vi "Revision Query.vi"(8 "error in (no error)":errorcluster, 11 "VISA resource name":refnum<visa-resource-name>) -> (0 "error out":errorcluster, 1 "Instrument Firmware Revision":string, 2 "Instrument Driver Revision":string, 3 "VISA resource name out":refnum<visa-resource-name>)   [LabVIEW 2025]
doc: "Queries the current instrument firmware revision and instrument driver revision.\n\nRefer to the Readme file for detailed driver information including modification history."
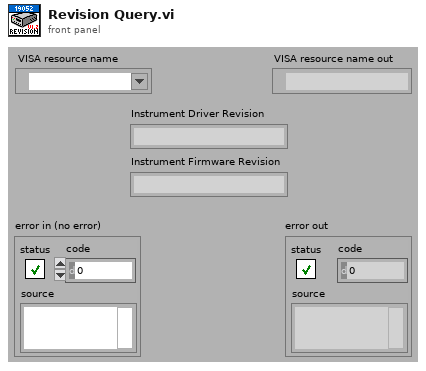
[diagram p1: front panel]
types:
  T1 = enum32{"invalid app kind", "Development System", "Run Time System", "Student Edition", "Embedded LabVIEW", "Evaluation", "Custom"}
  T2 = cluster{"Major":u16, "Minor":u16, "Fix":u16, "Build":u16}
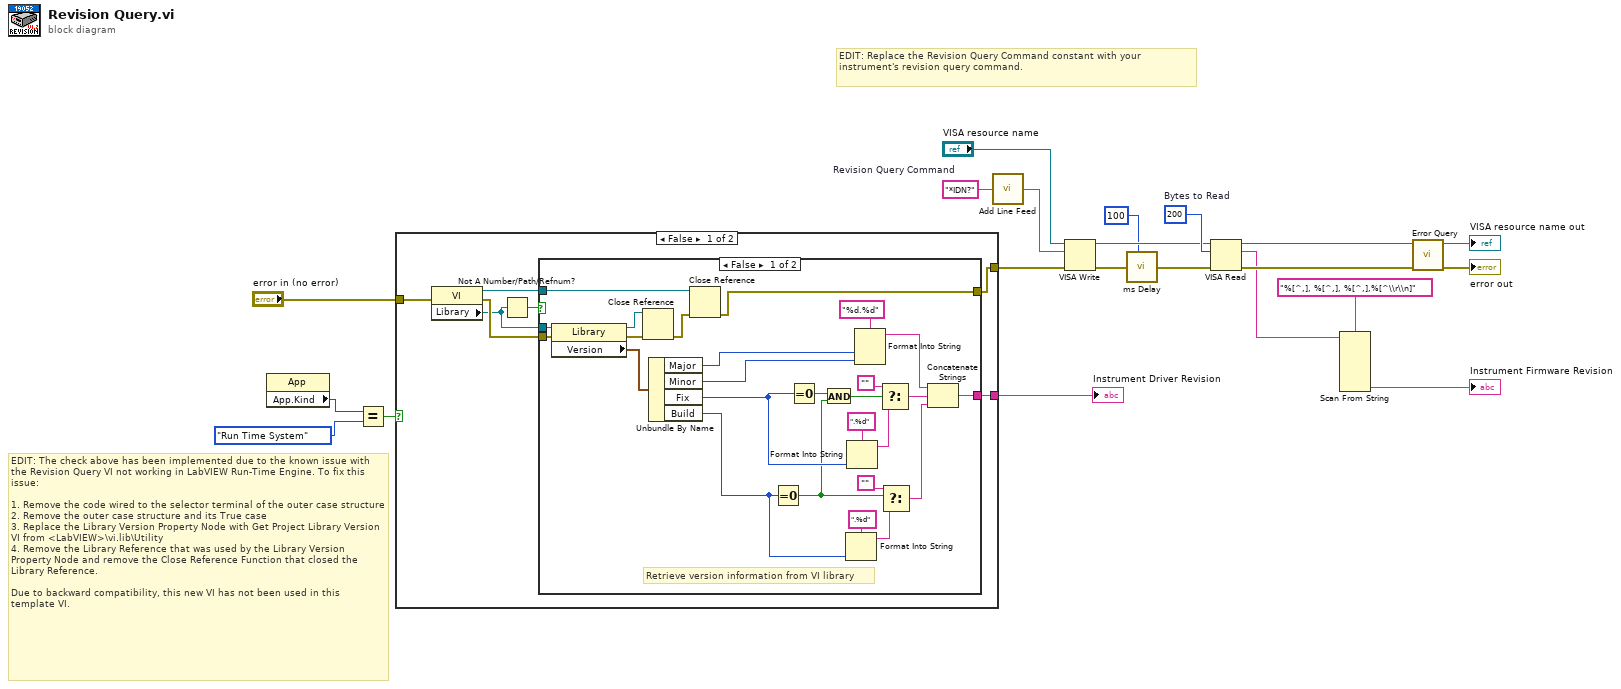
[diagram p0: block diagram]
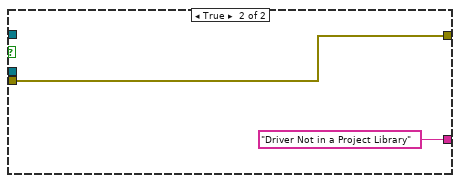
[diagram p2: hidden frame]
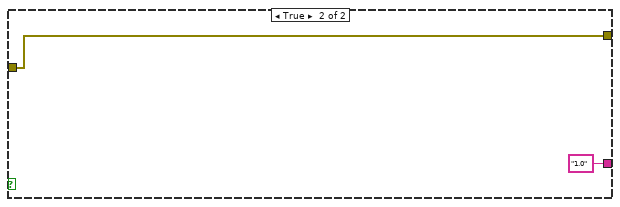
[diagram p3: hidden frame]
diagram:
  w5 = "*IDN?"  # Revision Query Command
  w18 = u32 200  # Bytes to Read
  # "EDIT: The check above has been implemented due to the known issue with the Revision Query VI not working in LabVIEW Run-Time Engine. To fix this issue:\n\n1. Remove the code wired to the selector terminal of the outer case structure\n2. Remove the outer case structure and its True case\n3. Replace the Library Version Property Node with Get Project Library Version VI from <LabVIEW>\\vi.lib\\Utility\n4. Remove the Library Reference that was used by the Library Version Property Node and remove the Close Reference Function that closed the Library Reference.\n\nDue to backward compatibility, this new VI has not been used in this template VI."
  # "EDIT: Replace the Revision Query Command constant with your instrument's revision query command."
  n1 = property class="App"() -> ("App.Kind"=w7:T1)  [unwired: 2 in, 2 out]
  n2 = Equal?(x=w7, y=T1."Run Time System" ("Application:Kind")) -> (x = y?=w8:bool)
  n3 = case shown="False" w8 {
    tunnel: [w24 "1.0"] -> w11
    tunnel: "error in (no error)" -> [w23 w57]
    tunnel: [w22 w57] -> w9
    frame False {
      n4 = property class="VI"(error in=w23) -> (reference out=w28:refnum<vi>, error out=w27:errorcluster, "Library"=w26:refnum<vi>)  [unwired: 1 in]
      n5 = Not A Number/Path/Refnum?(number/path/refnum=w26) -> (NaN/Path/Refnum?=w25:bool)
      n6 = case shown="False" w25 {
        tunnel: w28 -> [w51 _]
        tunnel: w27 -> [w36 w56]
        tunnel: [w31 w56] -> w22
        tunnel: [w30 "Driver Not in a Project Library"] -> w24
        tunnel: w26 -> [w29 _]
        frame False {
          # "Retrieve version information from VI library"
          n7 = property class="Library"(reference=w29, error in=w36) -> (reference out=w53:refnum<vi>, error out=w54:errorcluster, "Version"=w50:T2)
          n8 = Close Reference(reference=w53, error in (no error)=w54) -> (error out=w52:errorcluster)
          n9 = Unbundle By Name(w50) -> ("Major"=w39:u16, "Minor"=w38:u16, "Fix"=w35:u16, "Build"=w37:u16)
          n10 = Close Reference(reference=w51, error in (no error)=w52) -> (error out=w31:errorcluster)
          n11 = Equal To 0?(x=w37) -> (x = 0?=w33:bool)
          n12 = Equal To 0?(x=w35) -> (x = 0?=w34:bool)
          n13 = And(x=w34, y=w33) -> (x .and. y?=w32:bool)
          n14 = Format Into String(format string=".%d", w37) -> (resulting string=w43:string)  [unwired: 2 in, 1 out]
          n15 = Format Into String(format string=".%d", w35) -> (resulting string=w47:string)  [unwired: 2 in, 1 out]
          n16 = Format Into String(format string="%d.%d", w39, w38) -> (resulting string=w45:string)  [unwired: 2 in, 1 out]
          n17 = Select(t="", s=w32, f=w47) -> (s? t:f=w44:string)
          n18 = Select(t="", s=w33, f=w43) -> (s? t:f=w40:string)
          n19 = Concatenate Strings(w45, w44, w40) -> (w30:string)
        }
        frame True {
        }
      }
    }
    frame True {
    }
  }
  "Instrument Driver Revision" <- w11
  n20 = call <instrlib>:"Add Line Feed.vi"("Command string"=w5) -> ("Concatenated string"=w4:string)  [unwired: 4 in]
  n21 = VISA Write(VISA resource name="VISA resource name", write buffer=w4, error in (no error)=w9) -> (VISA resource name out=w17:refnum<visa-resource-name>, error out=w3:errorcluster)  [unwired: 1 out]
  n22 = call <instrlib>:"ms Delay.vi"("miliseconds to wait"=u32 100, "error in (no error)"=w3) -> ("error out"=w2:errorcluster)  [unwired: 6 in, 1 out]
  n23 = VISA Read(VISA resource name=w17, byte count=w18, error in (no error)=w2) -> (VISA resource name out=w14:refnum<visa-resource-name>, read buffer=w16:string, error out=w21:errorcluster)  [unwired: 1 out]
  n24 = Scan From String(format string="%[^,], %[^,], %[^,],%[^\\r\\n]", input string=w16) -> (output 4=→"Instrument Firmware Revision":string)  [unwired: 9 in, 3 out]
  n25 = call <instrlib>:"Error Query.vi"("error in (no error)"=w21, "VISA resource name"=w14) -> ("error out"=→"error out":errorcluster, "VISA resource name out"=→"VISA resource name out":refnum<visa-resource-name>)  [unwired: 6 in, 2 out]
